vi "Setup.vi"(9 "Active Project":refnum<vi>, 10 "NI.LV.Dialog Instance":refnum<vi>) -> (2 "Target":string, 3 "Script out":refnum<class "_Rename.lvclass">)   [LabVIEW 2025, in "_Rename.lvlib" / "_Rename.lvclass"]
uses:
  _Rename.lvclass
  _Rename.lvclass/_Rename.ctl
  _Shared/Project Stuff/Project Stuff.lvclass
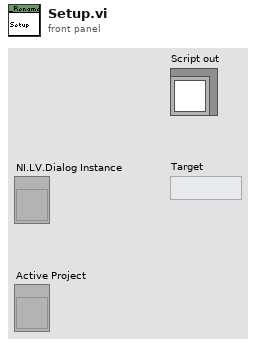
[diagram p1: front panel]
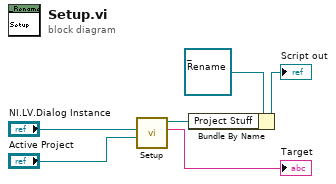
[diagram p0: block diagram]
diagram:
  n1 = call "Setup.vi"("Active Project"="Active Project", "NI.LV.Dialog Instance"="NI.LV.Dialog Instance") -> ("Target"=→"Target":string, "Project Stuff out"=w4:refnum<class "Project Stuff.lvclass">)  [unwired: 8 in]
  n2 = Bundle By Name(cluster=refnum<class "_Rename.lvclass"> refnum ("Script out"), "Project Stuff"=w4) -> (→"Script out":refnum<class "_Rename.lvclass">)
